vi "Gate Mode.vi"(7 "Read Value? (F)":bool, 8 "error in (no error)":errorcluster, 9 "Gate Mode (CW)":T1, 10 "Gate (A)":T2, 11 "VISA resource name":refnum<visa-resource-name>) -> (0 "error out":errorcluster, 1 "Gate Mode":T1, 3 "VISA resource name out":refnum<visa-resource-name>)   [LabVIEW 2013, in "SRS SR400.lvlib"]
doc: "<B>GM i { ,j }</B>\n\nThe GM command sets and reads the gate modes. i = 0 or 1 designates A gate or B gate and is required. If j is included, the selected gate is set to CW, j=0, or FIXED, j=1, or SCAN, j=2. If j is absent, the mode of gate i is returned. The mode may be changed during a scan. If it is changed to SCAN, the delay begins scanning from the start position on the next count period. If it is changed to FIXED, the delay returns to the start position immediately. If it is changed to CW, the gate immediately changes to continuously on."
uses:
  <instrlib>/SRS SR400/SRS SR400.lvlib
  <instrlib>/SRS SR400/Public/Typedefs/Gate.ctl
  <instrlib>/SRS SR400/Public/Typedefs/Gate Mode.ctl
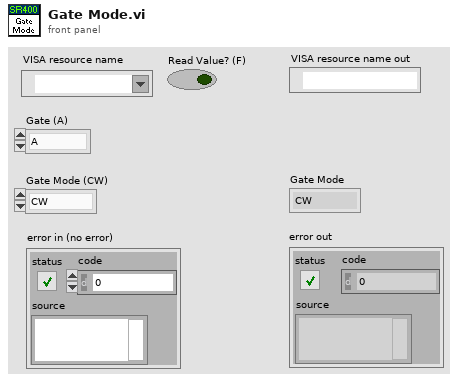
[diagram p1: front panel]
types:
  T1 = typedef "SRS SR400.lvlib/Gate Mode.ctl" = enum16{"CW", "Fixed", "Scan"}
  T2 = typedef "SRS SR400.lvlib/Gate.ctl" = enum16{"A", "B"}
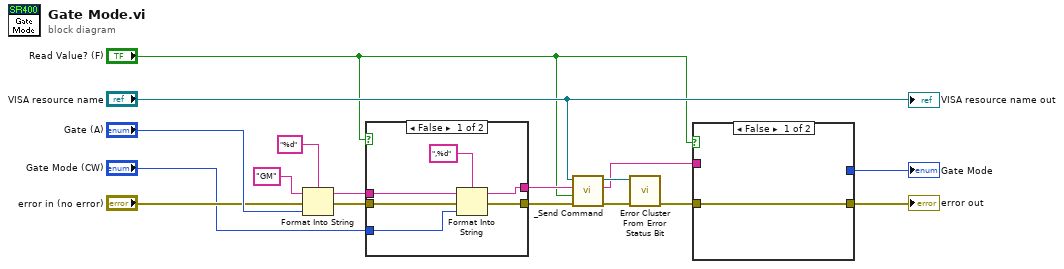
[diagram p0: block diagram]
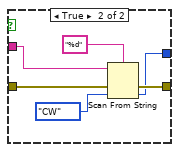
[diagram p2: hidden frame]
diagram:
  n1 = Format Into String(format string="%d", initial string="GM" ("command"), error in="error in (no error)", "Gate (A)") -> (resulting string=w14:string, error out=w15:errorcluster)
  n2 = case shown="False" "Read Value? (F)" {
    tunnel: w15 -> [w23 w24]
    tunnel: w14 -> [w18 w25]
    tunnel: "Gate Mode (CW)" -> [w22 _]
    tunnel: [w20 w25] -> w10
    tunnel: [w19 w24] -> w9
    frame False {
      n3 = Format Into String(format string=",%d", initial string=w18, error in=w23, w22) -> (resulting string=w20:string, error out=w19:errorcluster)
    }
    frame True {
    }
  }
  n4 = call <instrlib>:"_Send Command.vi"("error in (no error)"=w9, "Read Value? (F)"="Read Value? (F)", "Command"=w10, "VISA resource name"="VISA resource name") -> ("error out"=w6:errorcluster, "Response"=w2:string, "VISA resource name out"=w7:refnum<visa-resource-name>)  [unwired: 5 out]
  n5 = call <instrlib>:"Error Cluster From Error Status Bit.vi"("error in (no error)"=w6, "VISA resource name"=w7) -> ("error out"=w5:errorcluster)  [unwired: 8 in, 1 out]
  n6 = case shown="False" "Read Value? (F)" {
    tunnel: w5 -> [w26 w31]
    tunnel: [w26 w30] -> w4
    tunnel: w2 -> [_ w29]
    tunnel: [_ w27] -> w1
    frame False {
    }
    frame True {
      n7 = Scan From String(format string="%d", input string=w29, error in=w31, default 1=Gate_Mode."CW" ("Gate Mode (CW)")) -> (error out=w30:errorcluster, output 1=w27:T1)  [unwired: 1 in, 2 out]
    }
  }
  "error out" <- w4
  "Gate Mode" <- w1
  "VISA resource name out" <- "VISA resource name"
